vi "AuMT8852B Check Hex Byte String Value.vi"(5 "Number of bytes (6)":i32=6, 7 "Set/Get (Set)":enum16{"Set", "Get"}(ring), 8 "error in (no error)":errorcluster, 9 "Check IVI flag first? (T)":bool=TRUE, 10 "Hex byte string (0)":string="0", 11 "VISA session":refnum<visa-resource-name>) -> (0 "error out":errorcluster, 3 "VISA session out":refnum<visa-resource-name>, 4 "Hex byte string out":string)   [LabVIEW 2017]
doc: "Anritsu MT8852B Bluetooth Tester\n\nChecks and Coerces a string hex value to an appropriate length and value.\n\nINPUTS\nSet/Get - range checking will be skipped if this control is Get.\nUpper limit, lower limit - valid range for the value (the limits are also valid values).\nCheck IVI flag first? - if True, range checking will not be done if the IVI range-checking flag is off. If False, this VI will not check the IVI flag."
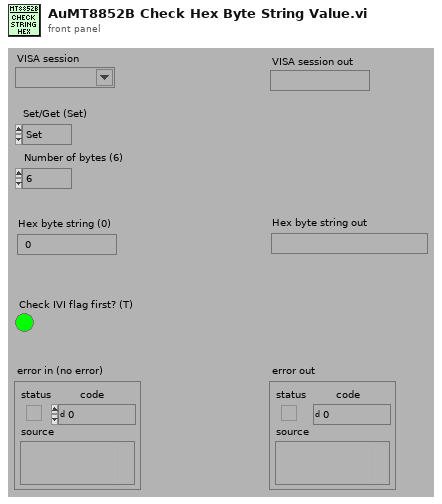
[diagram p1: front panel]
types:
  T1 = enum16{"Simulate", "Range check", "Cache", "Query instrument status"}
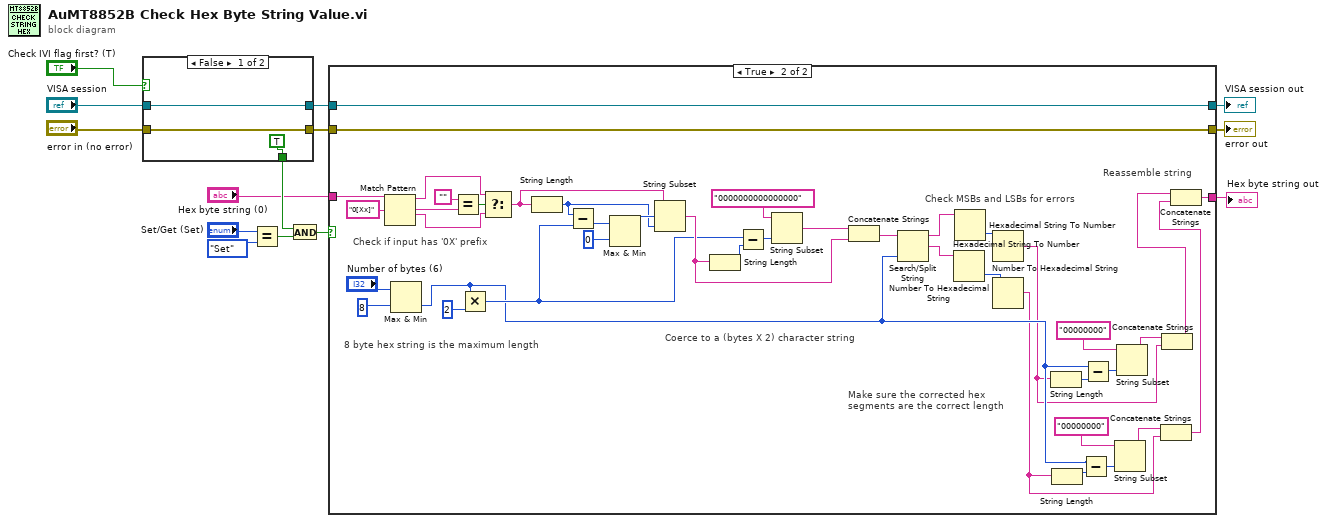
[diagram p0: block diagram]
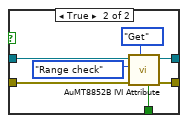
[diagram p2: hidden frame]
diagram:
  n1 = case shown="False" "Check IVI flag first? (T)" {
    tunnel: [w15 w24] -> w12
    tunnel: [w16 w23] -> w11
    tunnel: "VISA session" -> [w15 w22]
    tunnel: "error in (no error)" -> [w16 w21]
    tunnel: [TRUE ("Value out") w18] -> w4
    frame False {
    }
    frame True {
      n2 = call <instrlib>:"AuMT8852B IVI Attribute.vi"("Set/Get (Set)"=enum16{"Set", "Get"}."Get", "error in (no error)"=w21, "Flag (Simulate)"=T1."Range check", "VISA session"=w22) -> ("error out"=w23:errorcluster, "VISA session out"=w24:refnum<visa-resource-name>, "Value out"=w18:bool)  [unwired: 5 in]
    }
  }
  n3 = Equal?(x="Set/Get (Set)", y=enum16{"Set", "Get"}."Set") -> (x = y?=w5:bool)
  n4 = And(x=w4, y=w5) -> (x .and. y?=w6:bool)
  n5 = case shown="True" w6 {
    tunnel: [w27 w69] -> w14
    tunnel: w12 -> [w27 w69]
    tunnel: [w26 w68] -> w13
    tunnel: w11 -> [w26 w68]
    tunnel: [w25 w46] -> w2
    tunnel: "Hex byte string (0)" -> [w25 w45]
    frame False {
    }
    frame True {
      # "Make sure the corrected hex \nsegments are the correct length"
      # "Reassemble string"
      # "Check MSBs and LSBs for errors"
      # "Coerce to a (bytes X 2) character string"
      # "Check if input has '0X' prefix"
      # "8 byte hex string is the maximum length"
      n6 = Match Pattern(string=w45, regular expression="0[Xx]") -> (before substring=w52:string, match substring=w51:string, after substring=w53:string)  [unwired: 1 in, 1 out]
      n7 = Max & Min(x="Number of bytes (6)", y=8) -> (min(x,y)=w34:i32)  [unwired: 1 out]
      n8 = Equal?(x="", y=w51) -> (x = y?=w49:bool)
      n9 = Multiply(x=w34, y=2) -> (x*y=w47:i32)
      n10 = Select(t=w52, s=w49, f=w53) -> (s? t:f=w65:string)
      n11 = String Length(string=w65) -> (length=w33:i32)
      n12 = Subtract(x=w33, y=w47) -> (x-y=w56:i32)
      n13 = Max & Min(x=w56, y=0) -> (max(x,y)=w57:i32)  [unwired: 1 out]
      n14 = String Subset(string=w65, offset (0)=w57, length (rest)=w33) -> (substring=w67:string)
      n15 = String Length(string=w67) -> (length=w61:i32)
      n16 = Subtract(x=w47, y=w61) -> (x-y=w62:i32)
      n17 = String Subset(string="0000000000000000", length (rest)=w62) -> (substring=w66:string)  [unwired: 1 in]
      n18 = Concatenate Strings(w66, w67) -> (w64:string)
      n19 = Search/Split String(string=w64, offset (0)=w34) -> (substring before match=w60:string, match + rest of string=w59:string)  [unwired: 1 in, 1 out]
      n20 = Hexadecimal String To Number(string=w59) -> (number=w58:u32)  [unwired: 2 in, 1 out]
      n21 = Hexadecimal String To Number(string=w60) -> (number=w54:u32)  [unwired: 2 in, 1 out]
      n22 = Number To Hexadecimal String(2:w54) -> (0:w29:string)  [unwired: 1 in]
      n23 = Number To Hexadecimal String(2:w58) -> (0:w31:string)  [unwired: 1 in]
      n24 = String Length(string=w29) -> (length=w44:i32)
      n25 = String Length(string=w31) -> (length=w39:i32)
      n26 = Subtract(x=w34, y=w39) -> (x-y=w40:i32)
      n27 = Subtract(x=w34, y=w44) -> (x-y=w43:i32)
      n28 = String Subset(string="00000000", length (rest)=w40) -> (substring=w30:string)  [unwired: 1 in]
      n29 = String Subset(string="00000000", length (rest)=w43) -> (substring=w28:string)  [unwired: 1 in]
      n30 = Concatenate Strings(w30, w31) -> (w37:string)
      n31 = Concatenate Strings(w28, w29) -> (w38:string)
      n32 = Concatenate Strings(w38, w37) -> (w46:string)
    }
  }
  "VISA session out" <- w14
  "error out" <- w13
  "Hex byte string out" <- w2
